vi "Publish Initialization Complete.vi"(8 "error in (no error)":errorcluster, 11 "Process in":refnum<class "Process.lvclass">) -> (0 "error out":errorcluster, 3 "Process out":refnum<class "Process.lvclass">)   [LabVIEW 2019, in "TimingDRV Engine.lvlib" / "Process.lvclass"]
uses:
  Process.lvclass
  Process.lvclass/Process.ctl
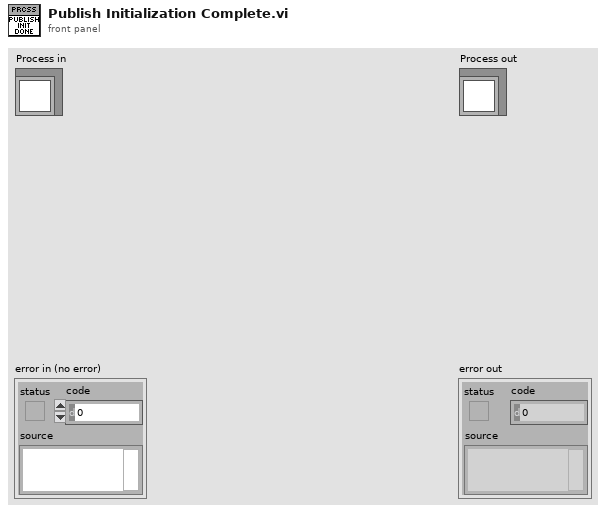
[diagram p1: front panel]
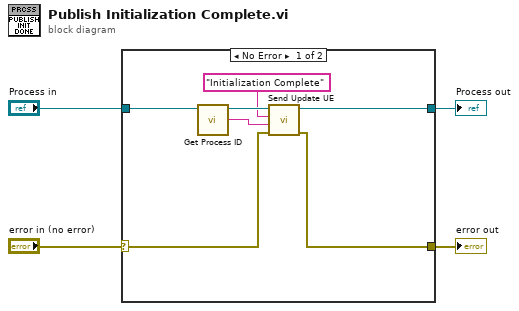
[diagram p0: block diagram]
diagram:
  n1 = case shown="No Error" "error in (no error)" {
    selector: "error in (no error)" -> [w8 w13]
    tunnel: [w7 w13] -> w3
    tunnel: [w9 w12] -> w1
    tunnel: "Process in" -> [w10 w12]
    frame No Error {
      n2 = call "Get Process ID.vi"("CD_Process in"=w10) -> ("Process ID"=w5:string, "CD_Process out"=w11:refnum<class "Process.lvclass">)  [unwired: 9 in]
      n3 = call "Send Update UE.vi"("error in (no error)"=w8, "Payload"=w5, "Update Message"="Initialization Complete" ("string"), "Process in"=w11) -> ("error out"=w7:errorcluster, "Process out"=w9:refnum<class "Process.lvclass">)  [unwired: 6 in]
    }
    frame Error {
    }
  }
  "error out" <- w3
  "Process out" <- w1
